vi "ParamNames_From_Captions.vi"(8 "error in":errorcluster, 10 "LV2011Compatbility":bool, 11 "captions":string[](array[string])) -> (0 "error out":errorcluster, 3 "Param Names":string[](array[string]))   [LabVIEW 2020]
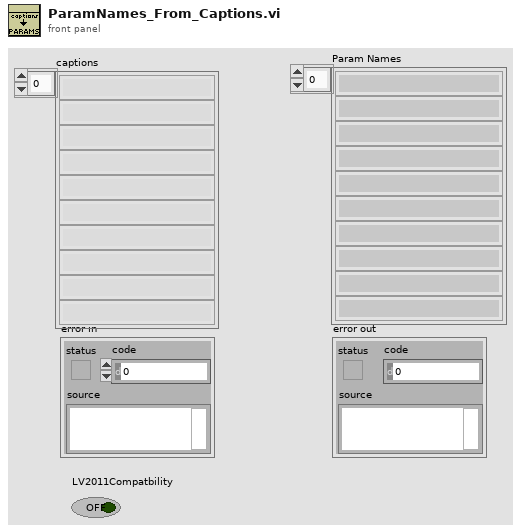
[diagram p1: front panel]
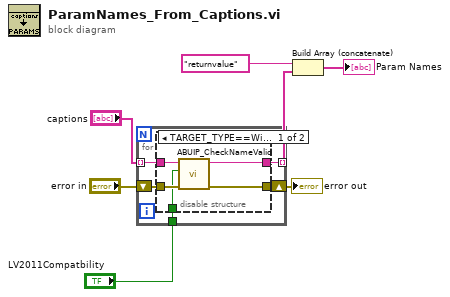
[diagram p0: block diagram]
diagram:
  n1 = for {
    tunnel: "captions" -> [w12] mode=indexing
    tunnel: [w11] -> w3 mode=indexing
    shift-right: [w9] -> w6
    shift-left: "error in" -> [w10]
    tunnel: "LV2011Compatbility" -> [w8]
    n2 = disable-structure shown="TARGET_TYPE==Windows" {
      disable-tunnel: w12 -> [w17 w18]
      disable-tunnel: [w16 w18] -> w11
      disable-tunnel: w10 -> [w15 _]
      disable-tunnel: [w14 _] -> w9
      disable-tunnel: w8 -> [w13 _]
      frame condition #0 (active) {
        n3 = call <resource>:"ABUIP_CheckNameValid.vi"("error in (no error)"=w15, "LV2011Compatibility"=w13, "name"=w17) -> ("error out"=w14:errorcluster, "valid name"=w16:string)  [unwired: 7 out]
      }
      frame condition #1 {
      }
    }
  }
  "error out" <- w6
  n4 = Build Array (concatenate)("returnvalue", w3) -> (→"Param Names":string[])
